vi "校准数据选择表.vi"(11 "量程下拉列表":enum16{"低量程", "高量程"}(ring)) -> (2 "布尔":bool=TRUE, 3 "ItemNames":string[](array[string]))   [LabVIEW 2016, in "斯坦道CODMn新电路板.lvlib"]
uses:
  <vilib>/Utility/miscctls.llb/LVPointTypeDef.ctl
panel:
  in  "确定":bool
  in  "返回":bool
  in  "数据表":T1
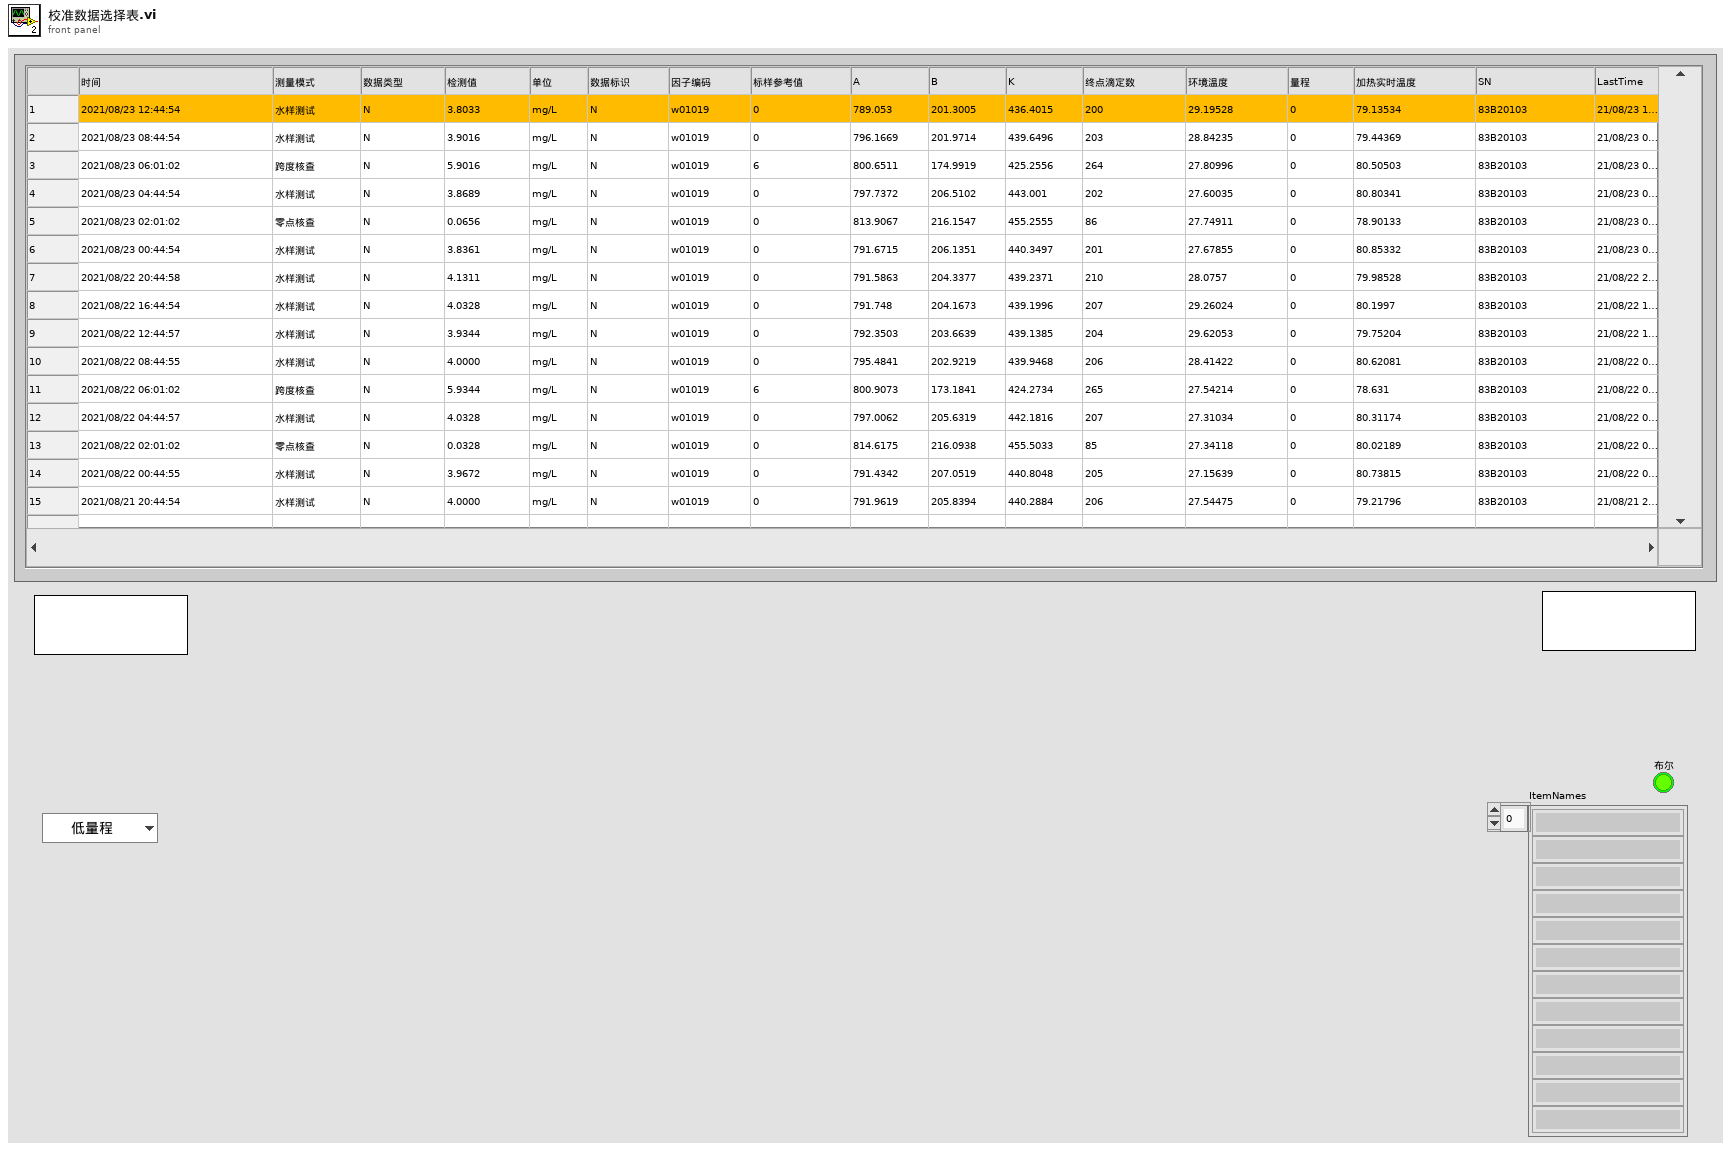
[diagram p1: front panel]
types:
  T1 = typedef "数据查询大列表框.ctl" = i32
  T2 = typedef "LVPointTypeDef.ctl" = cluster{"Horizontal":i16, "Vertical":i16}
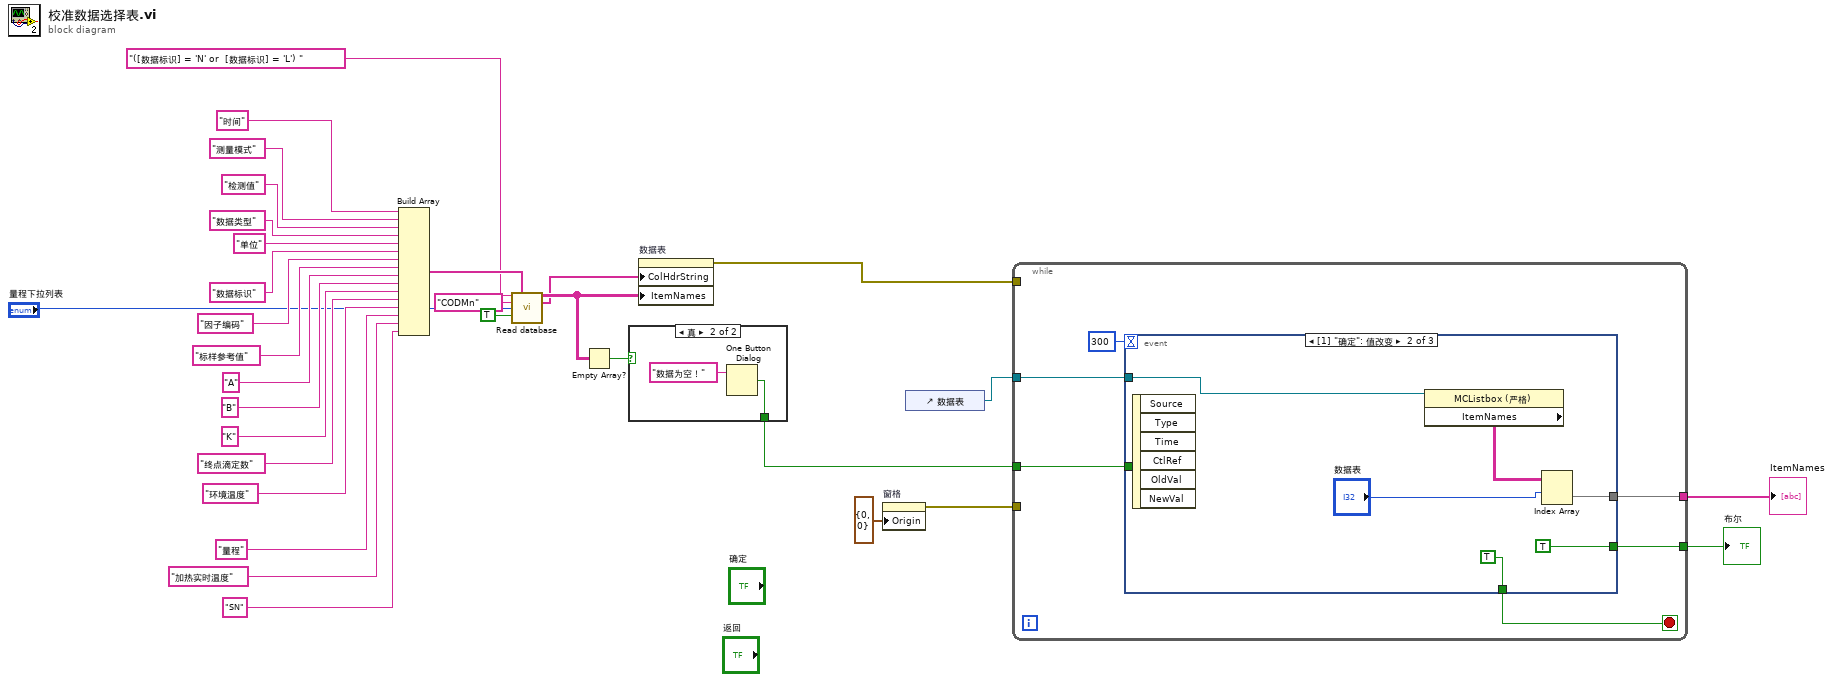
[diagram p0: block diagram]
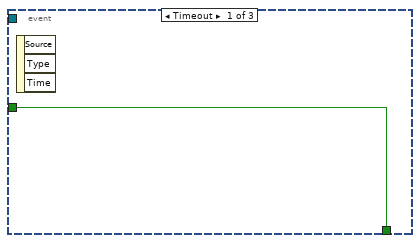
[diagram p3: hidden frame]
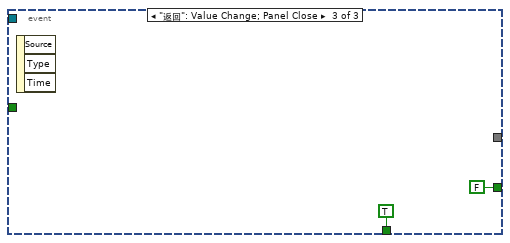
[diagram p4: hidden frame]
diagram:
  n1 = Build Array("时间", "测量模式", "检测值", "数据类型", "单位", "数据标识", "因子编码", "标样参考值", "A", "B", "K", "终点滴定数", "环境温度", "量程", "加热实时温度", "SN") -> (w15:string[])
  n2 = call "Read database.vi"("condition"="([数据标识] = 'N' or  [数据标识] = 'L') ", "显示项"=w15, "Table"="CODMn", "量程下拉列表"="量程下拉列表", "量程筛选"=TRUE) -> ("表格"=w26:string[][], "columns"=w1:string[])  [unwired: 6 in, 3 out]
  n3 = Empty Array?(array=w26) -> (empty?=w25:bool)
  n4 = case shown="真" w25 {
    tunnel: [_ w32] -> w24
    frame False {
    }
    frame True {
      n5 = One Button Dialog(message="数据为空！" ("消息")) -> (true=w32:bool)  [unwired: 1 in]
    }
  }
  n6 = property on="数据表" class="MCListbox (严格)"("ColHdrString"=w1, "ItemNames"=w26) -> (error out=w27:errorcluster)  [unwired: 2 in, 1 out]
  n7 = property on="窗格" class="Pane"("Origin"=T2 {"Horizontal"=0, "Vertical"=0} ("原点")) -> (error out=w29:errorcluster)  [unwired: 2 in, 1 out]
  n8 = control-ref of="数据表"() -> (w31:refnum<vi>)
  n9 = while {
    tunnel: w31 -> [w38]
    tunnel: [w37] -> w23
    tunnel: w29 -> [_]
    tunnel: [w36] -> w28
    tunnel: w27 -> [_]
    tunnel: w24 -> [w35]
    stop <- w39 stop-if-true
    n10 = event shown="[1] \"确定\": 值改变" {
      selector: _ -> [_ _ _]
      dyn-events: _ -> [_ _ _]
      timeout: 300 -> [_ _ _]
      tunnel: [w40 TRUE TRUE] -> w39
      tunnel: w38 -> [_ w43 _]
      tunnel: [_ w44 _] -> w37
      tunnel: [_ TRUE FALSE] -> w36
      tunnel: w35 -> [w40 _ _]
      event Timeout {
        n11 = event-data() -> ()  [unwired: 1 in, 3 out]
      }
      event "确定": Value Change {
        n12 = event-data() -> ()  [unwired: 1 in, 6 out]
        n13 = property class="MCListbox (严格)"(reference=w43) -> ("ItemNames"=w45:string[][])  [unwired: 1 in, 2 out]
        n14 = Index Array(array=w45, index (row)="数据表") -> (element=w44:string[])  [unwired: 1 in]
      }
      event "返回": Value Change; Panel Close {
        n15 = event-data() -> ()  [unwired: 1 in, 3 out]
      }
    }
  }
  "ItemNames" <- w23
  "布尔" <- w28
